vi "Wiimote Reset.vi"(8 "error in":errorcluster, 11 "hWiimoteHandle in":u32 format="%08x") -> (0 "error out":errorcluster, 3 "hWiimoteHandle out":u32 format="%08x")   [LabVIEW 2012, in "Wiimote.lvlib"]
uses:
  Wiimote.lvlib
  Wiimote LEDs.ctl
  Wiimote Reporting Mode.ctl
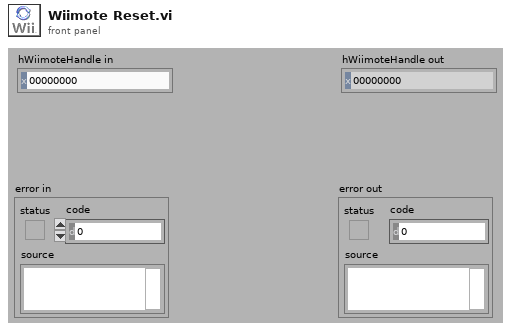
[diagram p1: front panel]
types:
  T1 = typedef "Wiimote.lvlib/Wiimote LEDs.ctl" = cluster{"LED 1":bool, "LED 2":bool, "LED 3":bool, "LED 4":bool}
  T2 = typedef "Wiimote.lvlib/Wiimote Reporting Mode.ctl" = u8
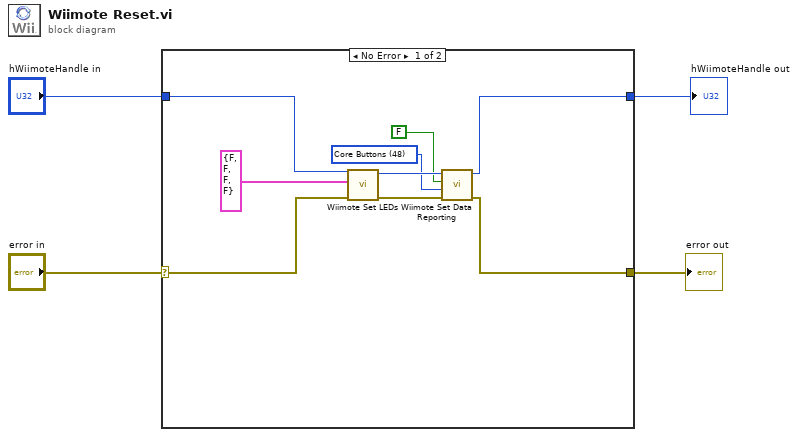
[diagram p0: block diagram]
diagram:
  n1 = case shown="No Error" "error in" {
    selector: "error in" -> [w12 w15]
    tunnel: [w7 w15] -> w3
    tunnel: "hWiimoteHandle in" -> [w13 w14]
    tunnel: [w8 w14] -> w1
    frame No Error {
      w5 = T2 48 items=["Status Information"=32, "Read Data"=33, "Write Data"=34, "Core Buttons"=48, "Core Buttons and Accelerometer"=49, "Core Buttons with 8 Extension bytes"=50, "Core Buttons and Accelerometer with 12 IR bytes"=51, "Core Buttons with 19 Extension bytes"=52, "Core Buttons and Accelerometer with 16 Extension Bytes"=53, "Core Buttons with 10 IR bytes and 9 Extension Bytes"=54, "Core Buttons and Accelerometer with 10 IR bytes and 6 Extension Bytes"=55] ("Reporting Mode")
      n2 = call "Wiimote Set LEDs.vi"("error in"=w12, "Wiimote LEDs"=T1 {"LED 1"=FALSE, "LED 2"=FALSE, "LED 3"=FALSE, "LED 4"=FALSE} ("Wiimote LEDs in"), "hWiimoteHandle in"=w13) -> ("error out"=w11:errorcluster, "hWiimoteHandle out"=w10:u32)  [unwired: 7 in]
      n3 = call "Wiimote Set Data Reporting.vi"("error in"=w11, "Reporting Mode"=w5, "Continuous"=FALSE, "hWiimoteHandle in"=w10) -> ("error out"=w7:errorcluster, "hWiimoteHandle out"=w8:u32)  [unwired: 6 in]
    }
    frame Error {
    }
  }
  "error out" <- w3
  "hWiimoteHandle out" <- w1
